vi "03Foot.vi"() -> ()   [LabVIEW 2020]
uses:
  <vilib>/DAQmx/read.llb/DAQmx Read (Digital 1D U8 1Chan NSamp).vi
  <vilib>/Instr/_visa.llb/VISA Configure Serial Port (Serial Instr).vi
  <vilib>/DAQmx/create/channels.llb/DAQmx Create Channel (DI-Digital Input).vi
  <vilib>/DAQmx/configure/timing.llb/DAQmx Timing (Change Detection).vi
  <vilib>/DAQmx/miscellaneous.llb/DAQmx Fill In Error Info.vi
  <vilib>/Utility/file.llb/Write Delimited Spreadsheet (I64).vi
panel:
  out "Array":T1(array[cluster])
  out "MPH READ":u8
  out "appended path":path
  out "Waveform Graph":dbl[](graph)
  out "String":string
  out "x-y":u32
  out "stopping":bool
  in  "lines":tag="cDAQ1Mod1/port0/line0"
  in  "Serial Port":refnum<visa-resource-name>="COM8"
  in  "stop":bool
  out "MPH":dbl min=0.0 max=12.0 step=0.1 format="%.1f"
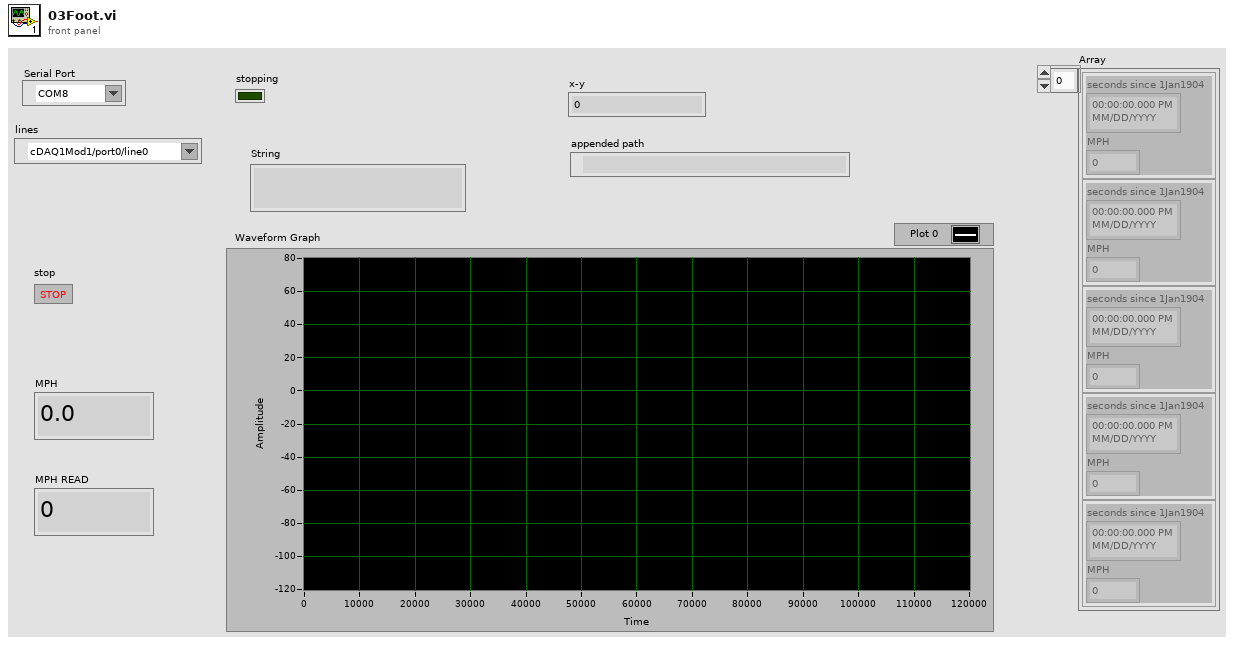
[diagram p1: front panel]
types:
  T1 = cluster{"seconds since 1Jan1904":timestamp, "MPH":dbl}[]
  T2 = enum16{"Initialize", "SetMPH", "GetData", "CheckTiming", "CompressWave", "StartDAQ", "StopDAQ"}
  T3 = enum16{"Initialize", "SetMPH", "GetData", "CheckTiming"}
  T4 = enum16{"Initialize", "SetMPH", "GetData", "CheckTiming", "CompressWave", "StartDAQ"}
  T5 = enum16{"Initialize", "SetMPH", "GetData", "CheckTiming", "CompressWave"}
  T6 = cluster{"seconds since 1Jan1904":timestamp, "MPH":dbl}
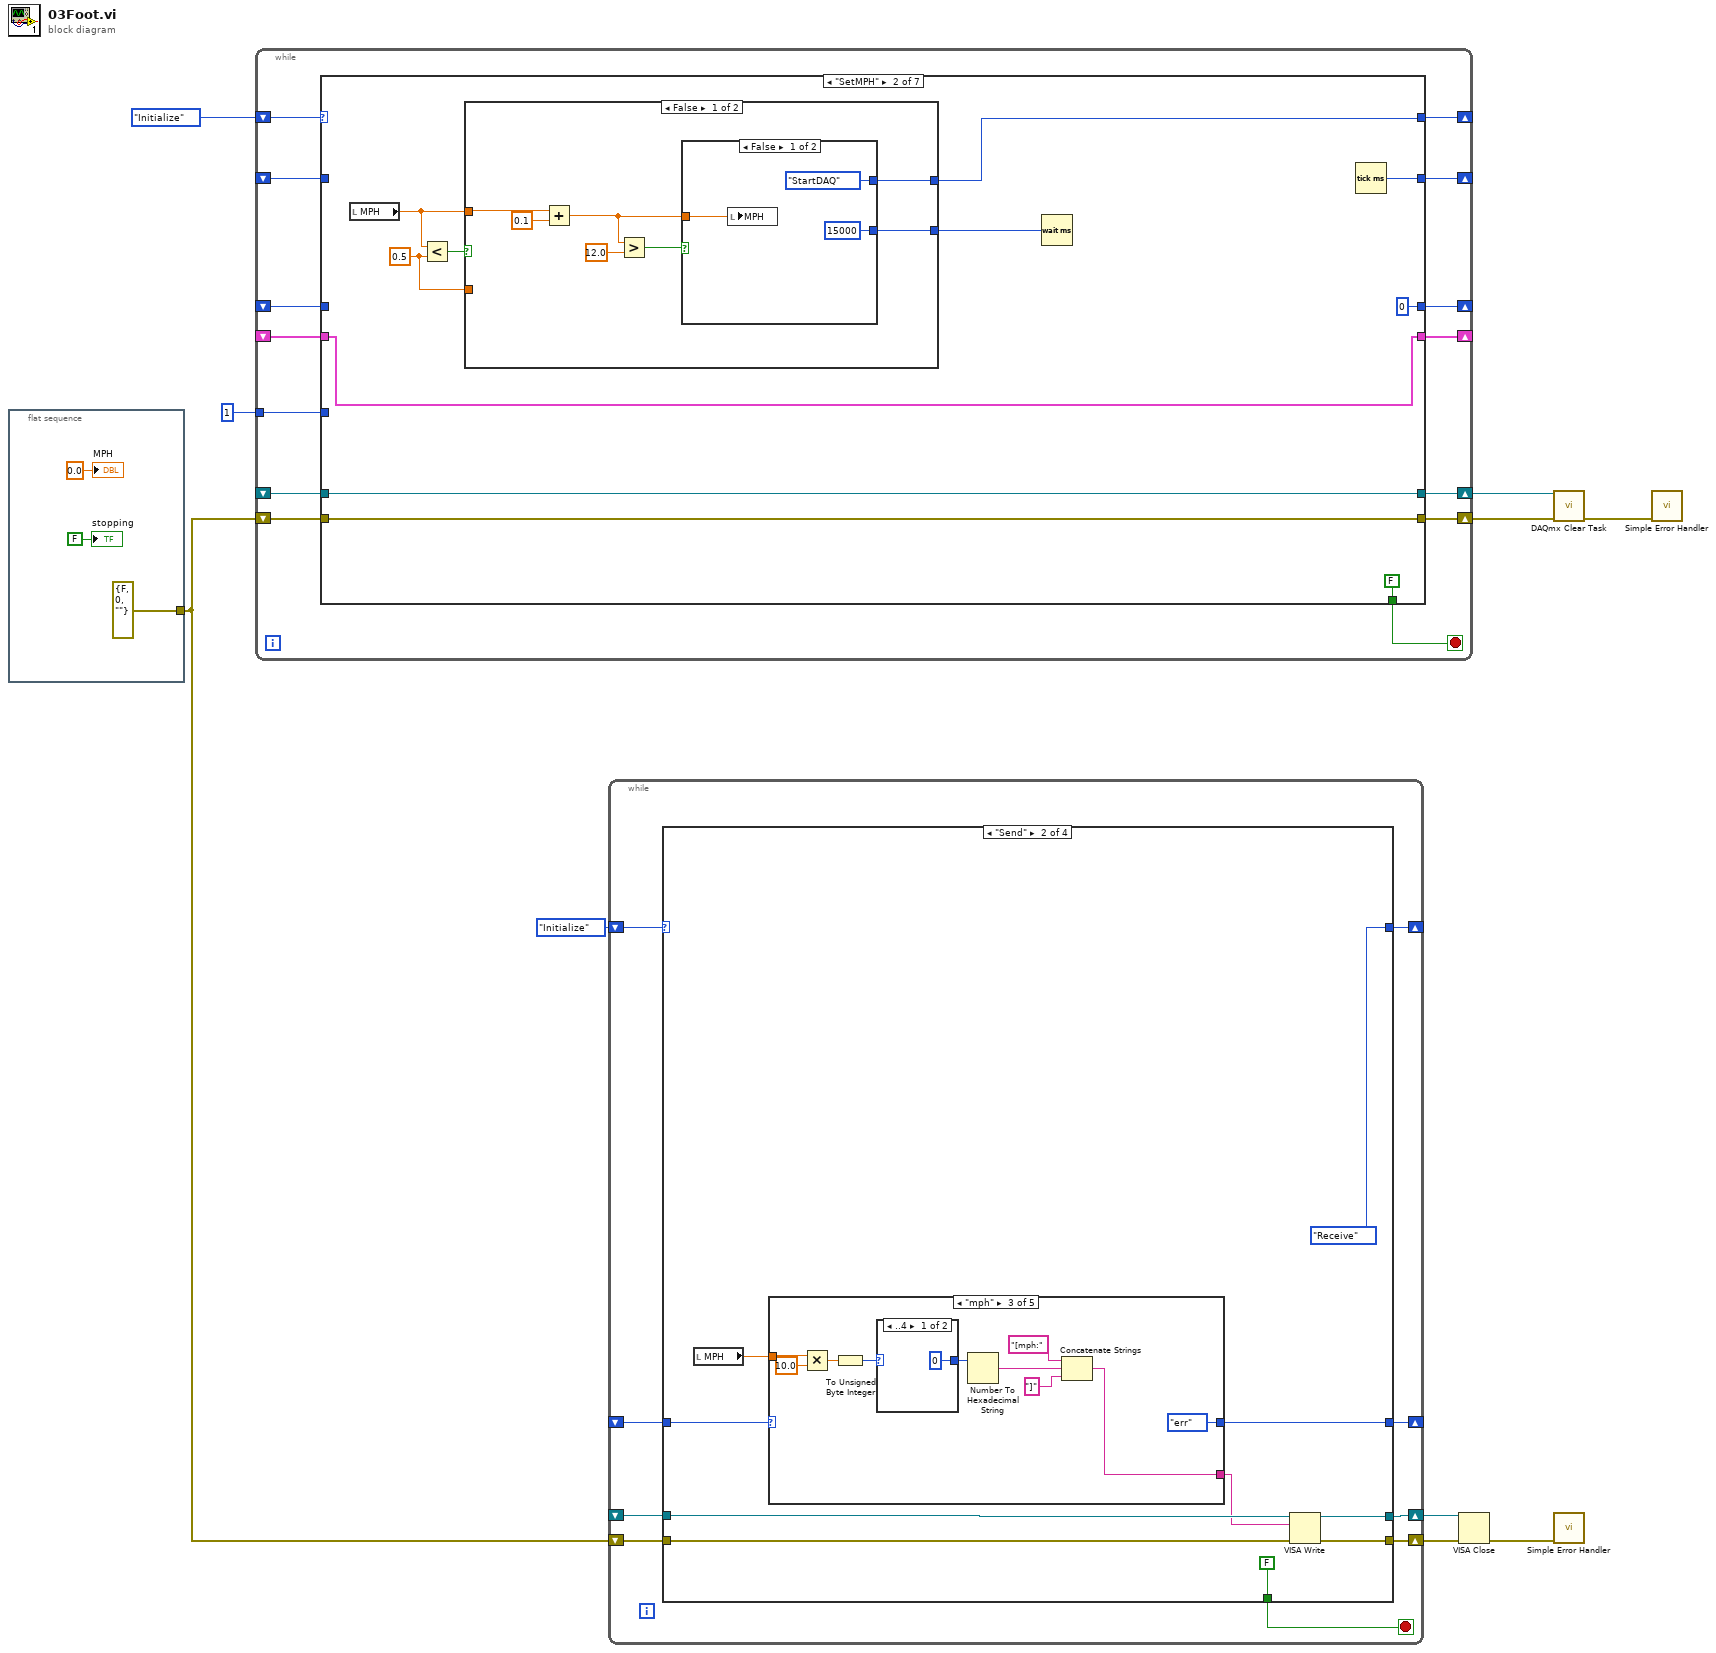
[diagram p0: block diagram]
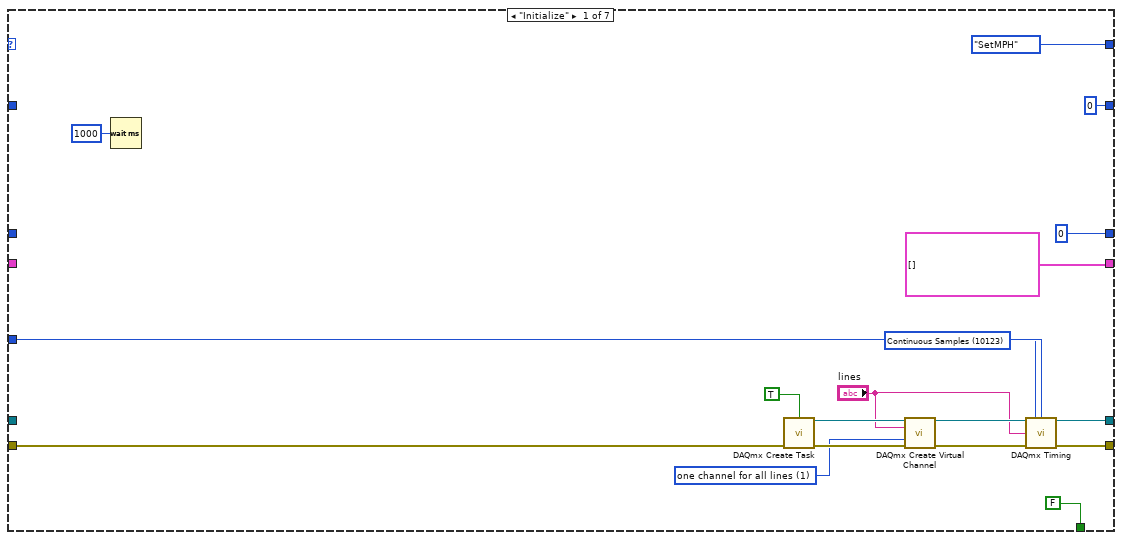
[diagram p2: hidden frame]
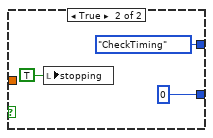
[diagram p3: hidden frame]
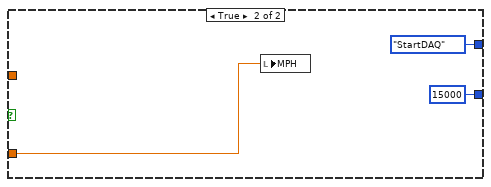
[diagram p4: hidden frame]
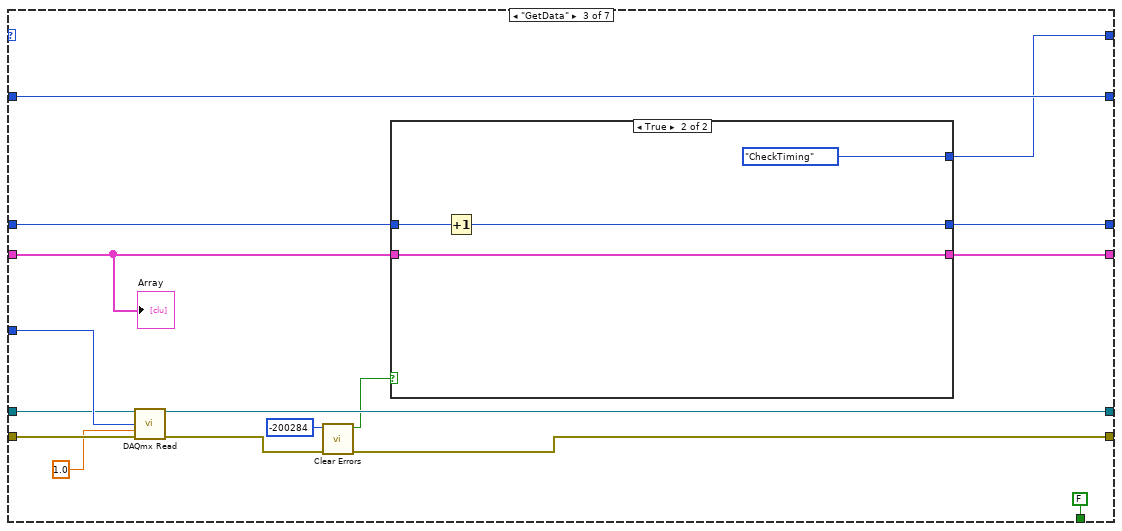
[diagram p5: hidden frame]
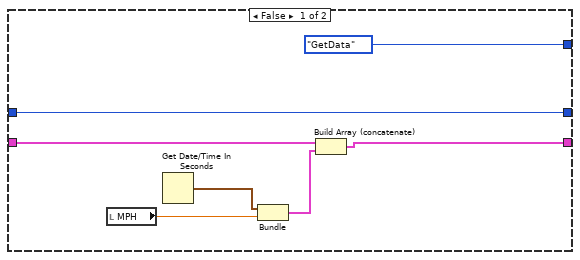
[diagram p6: hidden frame]
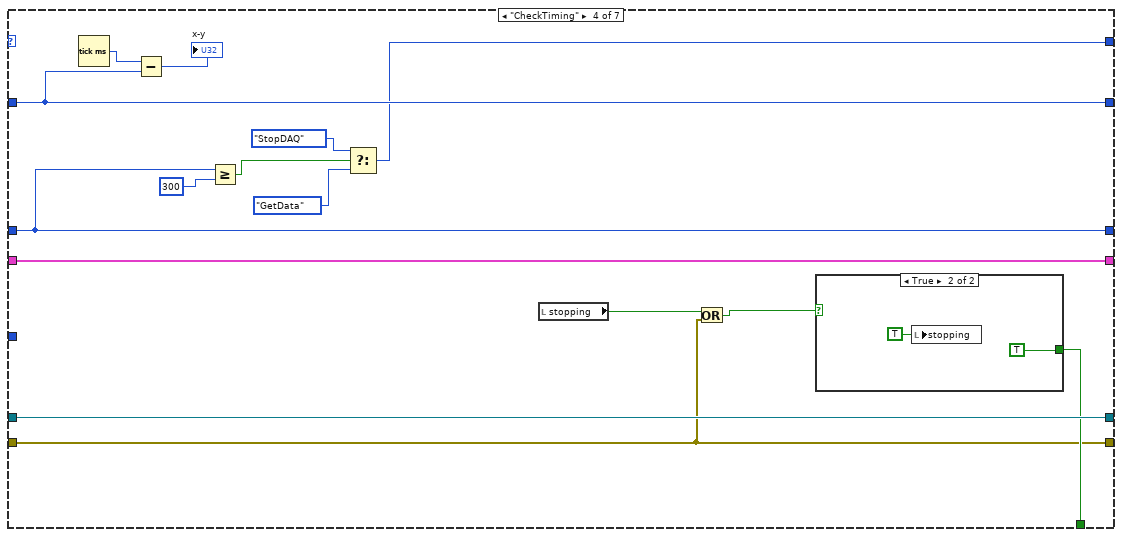
[diagram p7: hidden frame]
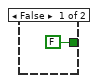
[diagram p8: hidden frame]
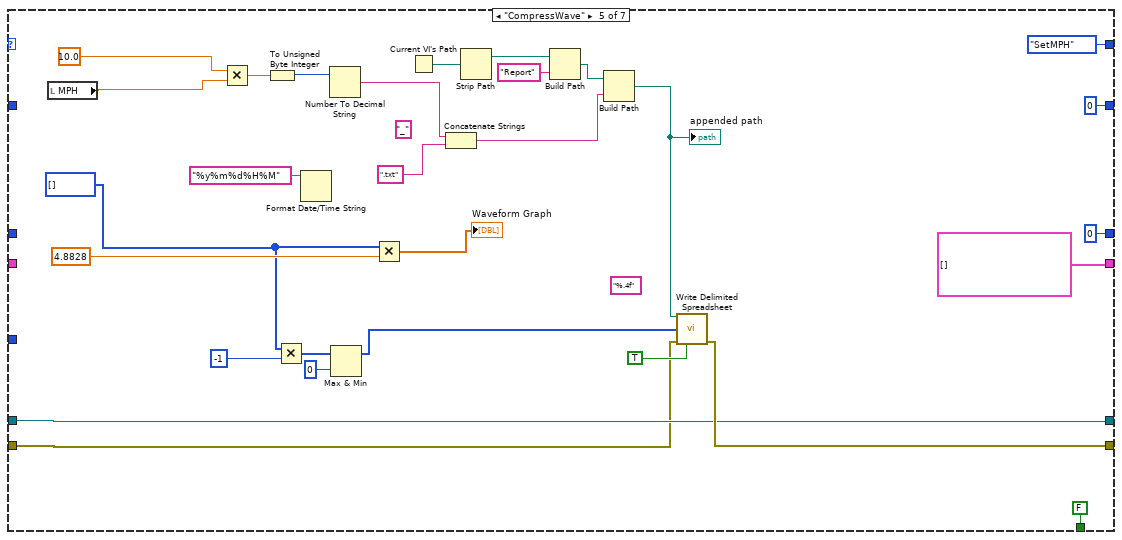
[diagram p9: hidden frame]
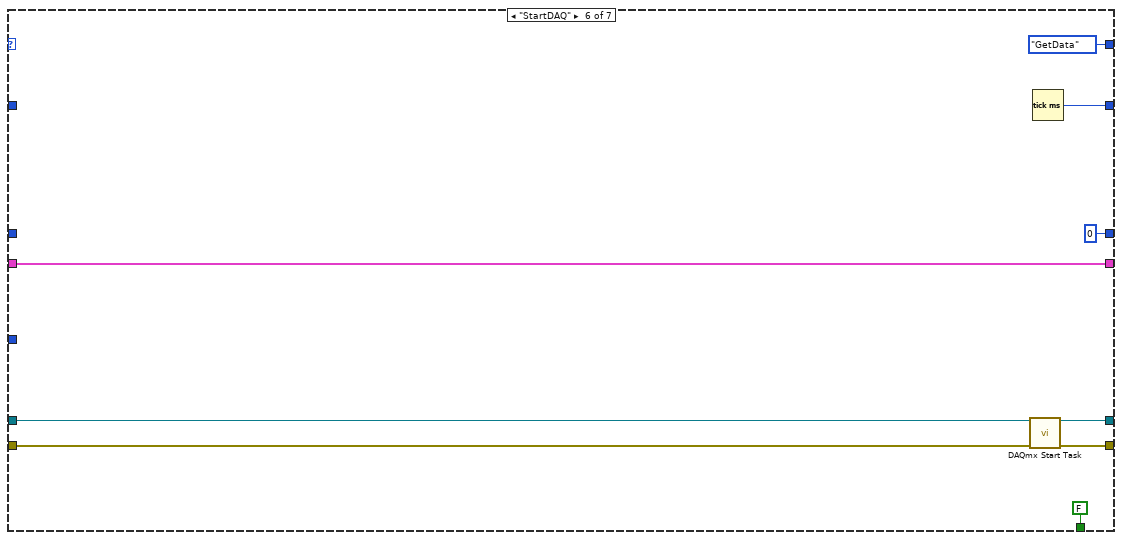
[diagram p10: hidden frame]
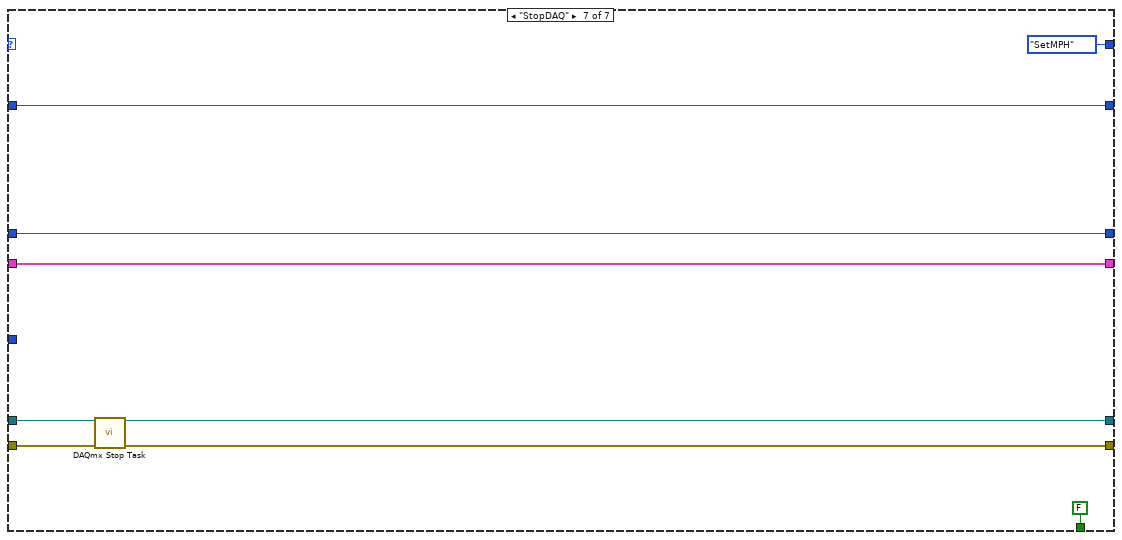
[diagram p11: hidden frame]
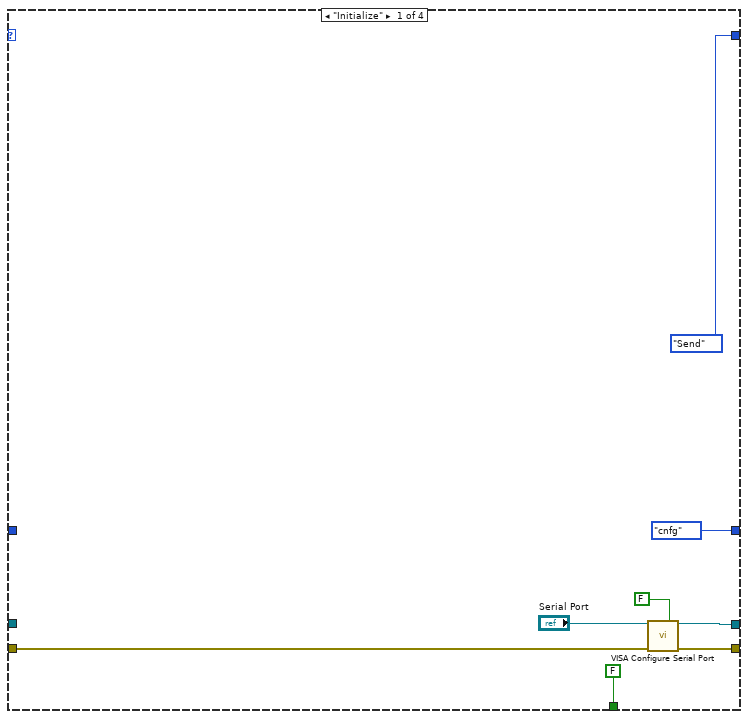
[diagram p12: hidden frame]
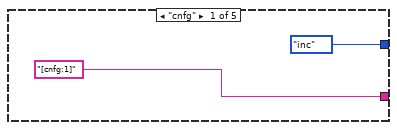
[diagram p13: hidden frame]
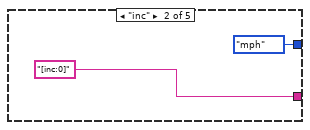
[diagram p14: hidden frame]
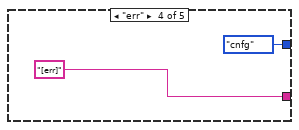
[diagram p16: hidden frame]
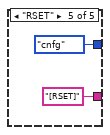
[diagram p17: hidden frame]
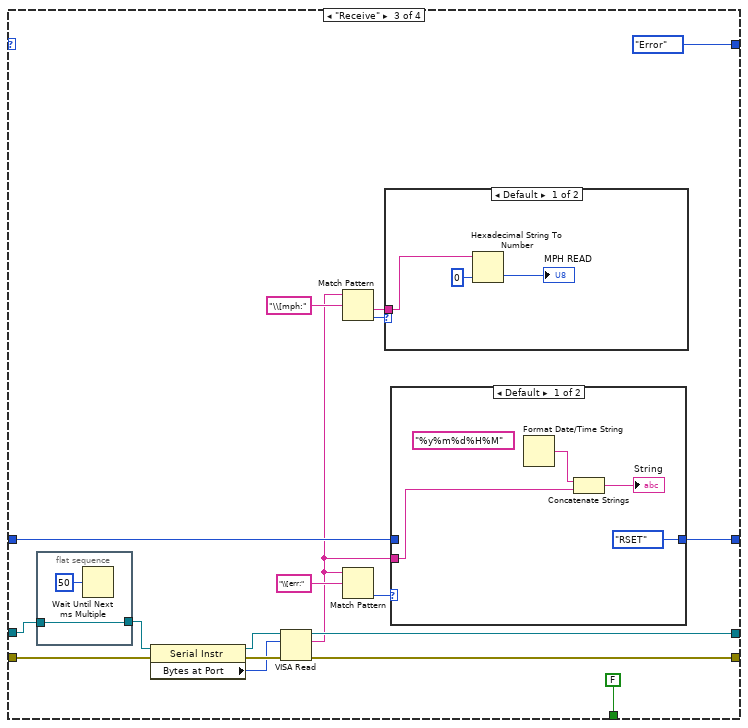
[diagram p18: hidden frame]
diagram:
  n1 = flat-sequence {
    tunnel: [errorcluster {"status"=FALSE, "code"=0, "source"=""} ("error constant")] -> w2
    frame #0 {
      "stopping" <- FALSE ("stopping")
      "MPH" <- 0.0 ("MPH")
    }
  }
  n2 = while {
    shift-right: [w26] -> _
    shift-left: T2."Initialize" -> [w27]
    shift-right: [w24] -> w4
    shift-left: _ -> [w22]
    shift-right: [w23] -> w5
    shift-left: w2 -> [w21]
    shift-right: [w20] -> _
    shift-left: _ -> [w19]
    tunnel: 1 ("samples per channel") -> [w18]
    shift-right: [w17] -> _
    shift-left: _ -> [w16]
    shift-right: [w15] -> _
    shift-left: _ -> [w14]
    stop <- w25 stop-if-true
    n3 = case shown="\"SetMPH\"" w27 {
      tunnel: [T3."SetMPH" w48 w77 w105 T5."SetMPH" T4."GetData" T2."SetMPH"] -> w26
      tunnel: [FALSE FALSE FALSE w111 FALSE FALSE FALSE] -> w25
      tunnel: [w35 w51 w85 w114 w122 w151 w160] -> w24
      tunnel: [w34 w50 w79 w107 w143 w152 w159] -> w23
      tunnel: w22 -> [_ w51 w84 w114 w122 w150 w162]
      tunnel: w21 -> [w31 w50 w83 w107 w121 w149 w161]
      tunnel: [u32 0 w49 w87 w110 u32 0 w154 w157] -> w20
      tunnel: w19 -> [_ _ w87 w110 _ _ w157]
      tunnel: w18 -> [w33 _ w86 _ _ _ _]
      tunnel: [u32 0 u32 0 w76 w102 u32 0 u32 0 w163] -> w17
      tunnel: w16 -> [_ _ w75 w102 _ _ w163]
      tunnel: [T1 [] w46 w74 w100 T1 [] w147 w156] -> w15
      tunnel: w14 -> [_ w46 w73 w100 _ w147 w156]
      frame "Initialize" {
        w32 = 10123 items=["Finite Samples"=10178, "Continuous Samples"=10123, "Hardware Timed Single Point"=12522] ("sample mode")
        w43 = 1 items=["one channel for each line", "one channel for all lines"] ("line grouping")
        n4 = Wait (ms)(milliseconds to wait=u32 1000) -> ()  [unwired: 1 out]
        n5 = call <vilib>:"DAQmx Create Task.vi"("auto cleanup"=TRUE, "error in"=w31) -> ("task out"=w45:refnum<k21>, "error out"=w44:errorcluster)  [unwired: 12 in]
        n6 = call-poly <vilib>:"DAQmx Create Virtual Channel.vi"("task in"=w45, "lines"="lines", "line grouping"=w43, "error in"=w44) -> ("task out"=w36:refnum<k21>, "error out"=w37:errorcluster)  [unwired: 10 in]
        n7 = call-poly <vilib>:"DAQmx Timing.vi"("task/channels in"=w36, "sample mode"=w32, "samples per channel"=w33, "rising edge physical channels"="lines", "error in"=w37) -> ("task out"=w35:refnum<k21>, "error out"=w34:errorcluster)  [unwired: 9 in]
      }
      frame "SetMPH" {
        w52 = 0.5 ("y")
        n8 = local read "MPH"() -> (w54:dbl)
        n9 = Less?(x=w54, y=w52) -> (x < y?=w55:bool)
        n10 = case shown="False" w55 {
          tunnel: w54 -> [w59 _]
          tunnel: [w61 u32 15000 ("milliseconds to wait")] -> w53
          tunnel: w52 -> [_ w71]
          tunnel: [w57 T4."StartDAQ"] -> w48
          frame False {
            n11 = Add(x=w59, y=0.1) -> (x+y=w58:dbl)
            n12 = Greater?(x=w58, y=12.0) -> (0:w62:bool)
            n13 = case shown="False" w62 {
              tunnel: w58 -> [w65 _]
              tunnel: [u32 15000 ("milliseconds to wait") u32 0 ("milliseconds to wait")] -> w61
              tunnel: [T4."StartDAQ" T4."CheckTiming"] -> w57
              frame False {
                n14 = local write "MPH"(w65) -> ()
              }
              frame True {
                n15 = local write "stopping"(TRUE ("stopping")) -> ()
              }
            }
          }
          frame True {
            n16 = local write "MPH"(w71) -> ()
          }
        }
        n17 = Wait (ms)(milliseconds to wait=w53) -> ()  [unwired: 1 out]
        n18 = Tick Count (ms)() -> (millisecond timer value=w49:u32)
      }
      frame "GetData" {
        n19 = call-poly <vilib>:"DAQmx Read.vi"("task/channels in"=w84, "number of samples per channel"=w86, "timeout"=1.0, "error in"=w83) -> ("task out"=w85:refnum<k21>, "error out"=w80:errorcluster)  [unwired: 9 in, 1 out]
        n20 = call <vilib>:"Clear Errors.vi"("error in (no error)"=w80, "specific error code to clear (0: all)"=-200284) -> ("error out"=w79:errorcluster, "specific error cleared?"=w78:bool)  [unwired: 4 in]
        n21 = case shown="True" w78 {
          tunnel: [T2."GetData" T2."CheckTiming"] -> w77
          tunnel: [w95 w97] -> w76
          tunnel: w75 -> [w95 w98]
          tunnel: [w90 w96] -> w74
          tunnel: w73 -> [w89 w96]
          frame False {
            n22 = local read "MPH"() -> (w91:dbl)
            n23 = Get Date/Time In Seconds() -> (seconds since 1Jan1904=w93:timestamp)
            n24 = Bundle("seconds since 1Jan1904"=w93, "MPH"=w91) -> (w92:T6)  [unwired: 1 in]
            n25 = Build Array (concatenate)(w89, w92) -> (w90:T1)
          }
          frame True {
            n26 = Increment(x=w98) -> (x+1=w97:u32)
          }
        }
        "Array" <- w73
      }
      frame "CheckTiming" {
        n27 = Tick Count (ms)() -> (millisecond timer value=w113:u32)
        n28 = Subtract(x=w113, y=w110) -> (x-y=→"x-y":u32)
        n29 = Greater Or Equal?(x=w102, y=u32 300) -> (x >= y?=w106:bool)
        n30 = Select(t=T2."StopDAQ", s=w106, f=T2."GetData") -> (s? t:f=w105:T2)
        n31 = local read "stopping"() -> (w109:bool)
        n32 = Or(x=w109, y=w107) -> (x .or. y?=w108:bool)
        n33 = case shown="True" w108 {
          tunnel: [FALSE TRUE] -> w111
          frame False {
          }
          frame True {
            n34 = local write "stopping"(TRUE ("stopping")) -> ()
          }
        }
      }
      frame "CompressWave" {
        w120 = i32[] []
        (unwired) "%.4f" ("format (%.3f)")
        (unwired) "_" ("string")
        n35 = local read "MPH"() -> (w127:dbl)
        n36 = Multiply(x=10.0, y=w127) -> (x*y=w132:dbl)
        n37 = To Unsigned Byte Integer(number=w132) -> (unsigned 8bit integer=w131:u8)
        n38 = Multiply(x=w120, y=-1) -> (x*y=w125:i32[])
        n39 = Format Date/Time String(time format string (%c)="%y%m%d%H%M") -> ()  [unwired: 2 in, 1 out]
        n40 = Number To Decimal String(number=w131) -> (decimal integer string=w130:string)  [unwired: 1 in]
        n41 = Max & Min(x=w125, y=0) -> (max(x,y)=w123:i32[])  [unwired: 1 out]
        n42 = Multiply(x=w120, y=4.8828) -> (x*y=→"Waveform Graph":dbl[])
        n43 = Current VI's Path() -> (path=w141:path)
        n44 = Concatenate Strings(w130, ".txt" ("string")) -> (w135:string)
        n45 = Strip Path(path=w141) -> (stripped path=w138:path)  [unwired: 1 out]
        n46 = Build Path(base path=w138, name or relative path="Report") -> (appended path=w136:path)
        n47 = Build Path(base path=w136, name or relative path=w135) -> (appended path=w134:path)
        "appended path" <- w134
        n48 = call-poly <vilib>:"Write Delimited Spreadsheet.vi"("file path (dialog if empty)"=w134, "1D data"=w123, "error in (no error)"=w121, "transpose? (no:F)"=TRUE ("transpose? (F)")) -> ("error out"=w143:errorcluster)  [unwired: 10 in, 1 out]
      }
      frame "StartDAQ" {
        n49 = call <vilib>:"DAQmx Start Task.vi"("task/channels in"=w150, "error in"=w149) -> ("task out"=w151:refnum<k21>, "error out"=w152:errorcluster)  [unwired: 12 in]
        n50 = Tick Count (ms)() -> (millisecond timer value=w154:u32)
      }
      frame "StopDAQ" {
        n51 = call <vilib>:"DAQmx Stop Task.vi"("task/channels in"=w162, "error in"=w161) -> ("task out"=w160:refnum<k21>, "error out"=w159:errorcluster)  [unwired: 12 in]
      }
    }
  }
  n52 = while {
    shift-right: [w169] -> w8
    shift-left: w2 -> [w173]
    shift-right: [w170] -> w9
    shift-left: _ -> [w172]
    shift-right: [w168] -> _
    shift-left: enum16{"Initialize", "Send", "Receive", "Error"}."Initialize" -> [w171]
    shift-right: [w167] -> _
    shift-left: _ -> [w166]
    stop <- w165 stop-if-true
    n53 = case shown="\"Send\"" w171 {
      tunnel: w173 -> [w177 w189 w225 w241]
      tunnel: w172 -> [_ w188 w224 w245]
      tunnel: [w179 w191 w223 w245] -> w170
      tunnel: [w178 w190 w216 w241] -> w169
      tunnel: [enum16{"Initialize", "Send", "Receive", "Error"}."Send" enum16{"Initialize", "Send", "Receive", "Error"}."Receive" enum16{"Initialize", "Send", "Receive", "Error"}."Error" enum16{"Initialize", "Send", "Receive", "Error"}."Send"] -> w168
      tunnel: [enum16{"cnfg", "inc", "mph", "err", "RSET"}."cnfg" w185 w218 w246] -> w167
      tunnel: w166 -> [_ w186 w217 w246]
      tunnel: [FALSE FALSE FALSE w240] -> w165
      frame "Initialize" {
        n54 = call-poly "VISA Configure Serial Port"("VISA resource name"="Serial Port", "Enable Termination\nChar (T)"=FALSE ("Enable Termination\nChar (T)"), "error in (no error)"=w177) -> ("VISA resource name out"=w179:refnum<visa-resource-name>, "error out"=w178:errorcluster)  [unwired: 11 in]
      }
      frame "Send" {
        n55 = local read "MPH"() -> (w182:dbl)
        n56 = case shown="\"mph\"" w186 {
          tunnel: ["[cnfg:1]" "[inc:0]" w196 "[err]" "[RSET]"] -> w187
          tunnel: w182 -> [_ _ w205 _ _]
          tunnel: [enum16{"cnfg", "inc", "mph", "err", "RSET"}."inc" enum16{"cnfg", "inc", "mph", "err", "RSET"}."mph" enum16{"cnfg", "inc", "mph", "err", "RSET"}."err" enum16{"cnfg", "inc", "mph", "err", "RSET"}."cnfg" enum16{"cnfg", "inc", "mph", "err", "RSET"}."cnfg"] -> w185
          frame "cnfg" {
          }
          frame "inc" {
          }
          frame "mph" {
            n57 = Multiply(x=w205, y=10.0) -> (x*y=w199:dbl)
            n58 = To Unsigned Byte Integer(number=w199) -> (unsigned 8bit integer=w198:u8)
            n59 = case shown="..4" w198 {
              selector: w198 -> [_ w207]
              tunnel: [u8 0 w207] -> w197
              frame ..4 {
              }
              frame 5.. {
              }
            }
            n60 = Number To Hexadecimal String(2:w197) -> (0:w202:string)  [unwired: 1 in]
            n61 = Concatenate Strings("[mph:" ("string"), w202, "]" ("string")) -> (w196:string)
          }
          frame "err" {
          }
          frame "RSET" {
          }
        }
        n62 = VISA Write(VISA resource name=w188, write buffer=w187, error in (no error)=w189) -> (VISA resource name out=w191:refnum<visa-resource-name>, error out=w190:errorcluster)  [unwired: 1 out]
      }
      frame "Receive" {
        n63 = flat-sequence {
          tunnel: w224 -> [w238]
          tunnel: [w238] -> w229
          frame #0 {
            n64 = Wait Until Next ms Multiple(millisecond multiple=u32 50) -> ()  [unwired: 1 out]
          }
        }
        n65 = property class="Serial Instr"(reference=w229, error in=w225) -> (reference out=w227:refnum<visa-resource-name>, error out=w228:errorcluster, "Bytes at Port"=w226:u32)
        n66 = VISA Read(VISA resource name=w227, byte count=w226, error in (no error)=w228) -> (VISA resource name out=w223:refnum<visa-resource-name>, read buffer=w214:string, error out=w216:errorcluster)  [unwired: 1 out]
        n67 = Match Pattern(string=w214, regular expression="\\[mph:") -> (after substring=w212:string, offset past match=w213:i32)  [unwired: 1 in, 2 out]
        n68 = Match Pattern(string=w214, regular expression="\\[err:") -> (offset past match=w219:i32)  [unwired: 1 in, 3 out]
        n69 = case shown="Default" w213 {
          tunnel: w212 -> [w232 _]
          frame Default {
            n70 = Hexadecimal String To Number(string=w232, default (0uL)=u8 0 ("default (0 I32)")) -> (number=→"MPH READ":u8)  [unwired: 1 in, 1 out]
          }
          frame -1 {
          }
        }
        n71 = case shown="Default" w219 {
          tunnel: [enum16{"cnfg", "inc", "mph", "err", "RSET"}."RSET" w237] -> w218
          tunnel: w217 -> [_ w237]
          tunnel: w214 -> [w233 _]
          frame Default {
            (unwired) "%y%m%d%H%M" ("time format string (%c)")
            n72 = Format Date/Time String() -> (date/time string=w234:string)  [unwired: 3 in]
            n73 = Concatenate Strings(w234, w233) -> (→"String":string)
          }
          frame -1 {
          }
        }
      }
      frame "Error" {
        n74 = local read "stopping"() -> (w242:bool)
        n75 = Compound Arithmetic op=OR("stop", w242, w241) -> (w244:bool)
        n76 = case shown="False" w244 {
          tunnel: [FALSE TRUE] -> w240
          frame False {
          }
          frame True {
            n77 = local write "stopping"(TRUE ("stopping")) -> ()
          }
        }
      }
    }
  }
  n78 = VISA Close(VISA resource name=w9, error in (no error)=w8) -> (error out=w7:errorcluster)
  n79 = call <vilib>:"DAQmx Clear Task.vi"("task in"=w4, "error in"=w5) -> ("error out"=w3:errorcluster)  [unwired: 13 in]
  n80 = call <vilib>:"Simple Error Handler.vi"("error in (no error)"=w7) -> ()  [unwired: 4 in, 5 out]
  n81 = call <vilib>:"Simple Error Handler.vi"("error in (no error)"=w3) -> ()  [unwired: 4 in, 5 out]
